vi "filename.vi"(11 "String":string) -> (3 "Path":path)   [LabVIEW 2015]
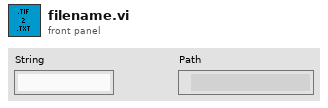
[diagram p1: front panel]
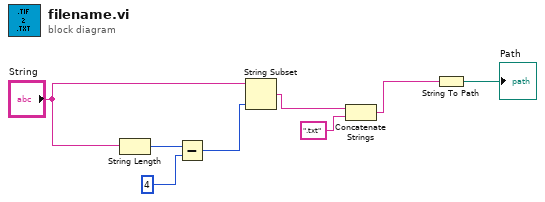
[diagram p0: block diagram]
diagram:
  n1 = String Length(string="String") -> (length=w7:i32)
  n2 = Subtract(x=w7, y=4) -> (x-y=w6:i32)
  n3 = String Subset(string="String", length (rest)=w6) -> (substring=w3:string)  [unwired: 1 in]
  n4 = Concatenate Strings(w3, ".txt") -> (w1:string)
  n5 = String To Path(string=w1) -> (path=→"Path":path)
